vi "APRSLogin.vi"(8 "error in (no error)":errorcluster, 11 "conRef":T1) -> (0 "error out":errorcluster, 3 "conRef out":T1)   [LabVIEW 2012]
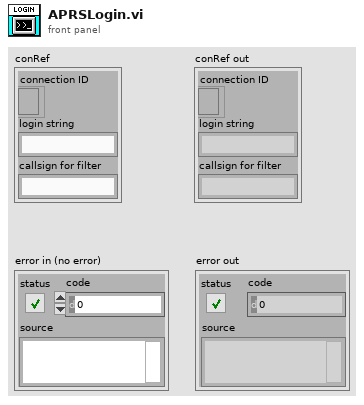
[diagram p1: front panel]
types:
  T1 = cluster{"connection ID":refnum<k5>, "login string":string, "callsign for filter":string}
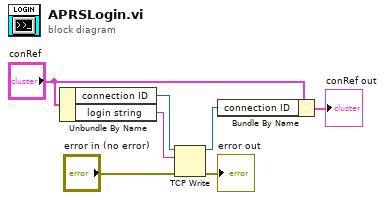
[diagram p0: block diagram]
diagram:
  n1 = Unbundle By Name("conRef") -> ("connection ID"=w5:refnum<k5>, "login string"=w4:string)
  n2 = TCP Write(connection ID=w5, data in=w4, error in (no error)="error in (no error)") -> (connection ID out=w2:refnum<k5>, error out=→"error out":errorcluster)  [unwired: 1 in, 1 out]
  n3 = Bundle By Name(cluster="conRef", "connection ID"=w2) -> (→"conRef out":T1)
